vi "GMLAN InitializeConnection.vi"(0 "CAN Interface":string(combo)="CAN1", 5 "Baudrate":u32, 7 "Transmit ID":u32, 9 "Receive ID":u32, 11 "error in (no error)":errorcluster, 12 "UUDT Receive ID":u32) -> (4 "UUDT Engine":T1, 6 "ADCS Ref":T2={"Diag CAN Handle"=0, "Transport Protocol"=enum."ISO TP - Normal Mode", "Receive Address Extension"=0, "Transmit Address Extension"=0, "Receive CAN Id"=0, "Transmit CAN Id"=0, "Log Frames ?"=FALSE, "My TP Address"=0, "Other TP Address"=0, "T1"=0, "T2"=0, "T3"=0, "T4"=0, "Tx SN"=0, "Block Size"=0, "Rx SN"=0, "VW TP Initialized?"=FALSE, "Tx block no"=0, "baud rate"=0, "Interface"="", "Channel Diag CAN Handle"=0, "UDP Connection ID"=refnum, "TCP Connection ID"=refnum, "Target IP Addr"=0, "Source Address"=0, "Target Address"=0, "Send Header NACK?"=FALSE, "DLL Handle"=0, "NAD"=0, "Time Stamp read first"=0.0, "Time Stamp read last"=0.0, "Time Stamp write first"=0.0, "Time Stamp write last"=0.0, "Time Stamp write"=0.0, "Time Stamp read"=0.0, " I/O Mode"=0, "FD Baudrate"=0, "TX_DL"=8, "RX_DL"=8, "DoIP Protocol Version"=1, " Selected I/O Mode"=0, "TesterPresent Counter"=0, "TesterPresent Limit"=0, "TesterPresent Tick[ms]"=10, "TesterPresent RequireResponse?"=FALSE, "TesterPresent Stored Ref?"=FALSE, "TesterPresent Message"=[], "TesterPresent Task Handle"=0, "TesterPresent Semaphore"=refnum, "Response Plausibility Check"=1, "Default Version?"=TRUE, "Diagostic Globals"={"Timeout FC (Bs)"=250, "Timeout CF (Cr)"=250, "Timeout Diag Command"=1000, "Receive Block Size (BS)"=0, "Wait Time CF (STmin)"=5, "Max Waits (N_WFTmax)"=10, "Waits to Send (N_WAIT)"=0, "Time between Waits (TW)"=25, "Fill CAN Frames?"=TRUE, "Fill Byte"=255, "Invalid Response as Error?"=FALSE, "Max RspPending Count"=5, "VWTP Command Timeout"=50, "Transport Protocol"=enum."Diagnostics on IP", "Diag CAN Handle"=0, "DLL Handle"=0, "Timeout RspPending"=1000}, "Session-based Properties?"=FALSE} {"Diagostic Globals"."Fill Byte" format="%x"; "TesterPresent Message" format="%.0x"; "Selected I/O Mode" items=["CAN", "CAN FD", "CAN FD+BRS", "ECU Determined"]; "DoIP Protocol Version" items=["2010"=1, "2012"=2]; "RX_DL" items=["8"=8, "12"=12, "16"=16, "20"=20, "24"=24, "32"=32, "48"=48, "64"=64]; "TX_DL" items=["8"=8, "12"=12, "16"=16, "20"=20, "24"=24, "32"=32, "48"=48, "64"=64]; "I/O Mode" items=["CAN", "CAN FD", "CAN FD+BRS", "Not yet determined"]}, 15 "error out":errorcluster)   [LabVIEW 2019, in "GMLAN.lvlib"]
uses:
  GMLAN.lvlib
  <vilib>/Automotive Diagnostic Command Set/Diagnostic Transport.llb/Diag Reference.ctl
  <vilib>/Automotive Diagnostic Command Set/Diagnostic Transport.llb/Transport Protocol Selector.ctl
  <vilib>/Automotive Diagnostic Command Set/Diagnostic Transport.llb/DoIP Protocol Version.ctl
  <vilib>/Automotive Diagnostic Command Set/Diagnostic Transport.llb/Diag Globals.ctl
  _Types/UUDT Engine Refs.ctl
  _Types/UUDT Engine Connection List_Action.ctl
  <vilib>/xnet/xnet.llb/XNET Create Session (Frame Input Queued).vi
  <vilib>/addons/Automotive Diagnostic Command Set/NI_Automotive Diagnostic Command Set.lvlib
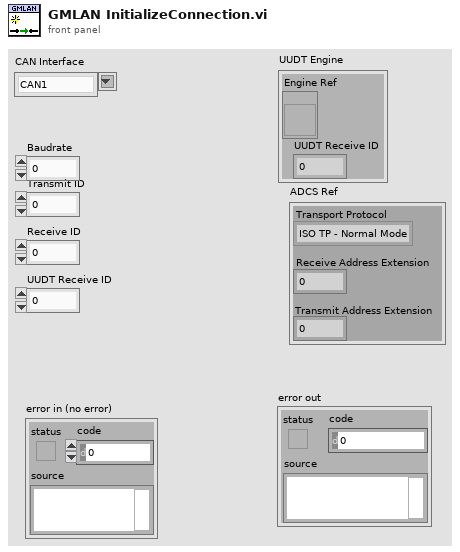
[diagram p1: front panel]
types:
  T1 = typedef "GMLAN.lvlib/UUDT Engine Refs.ctl" = cluster{"Engine Ref":refnum<vi>, "UUDT Receive ID":u32}
  T2 = typedef "NI_Automotive Diagnostic Command Set.lvlib/Diag Reference.ctl" = cluster{"Diag CAN Handle":u32, "Transport Protocol":T3, "Receive Address Extension":u8, "Transmit Address Extension":u8, "Receive CAN Id":u32, "Transmit CAN Id":u32, "Log Frames ?":bool, "My TP Address":u8, "Other TP Address":u8, "T1":u16, "T2":u16, "T3":u16, "T4":u16, "Tx SN":u8, "Block Size":u8, "Rx SN":u8, "VW TP Initialized?":bool, "Tx block no":u8, "baud rate":u64, "Interface":string, "Channel Diag CAN Handle":u32, "UDP Connection ID":refnum<k16>, "TCP Connection ID":refnum<k5>, "Target IP Addr":u32, "Source Address":u16, "Target Address":u16, "Send Header NACK?":bool, "DLL Handle":u32, "NAD":u8, "Time Stamp read first":dbl, "Time Stamp read last":dbl, "Time Stamp write first":dbl, "Time Stamp write last":dbl, "Time Stamp write":dbl, "Time Stamp read":dbl, " I/O Mode":u32, "FD Baudrate":u64, "TX_DL":u16, "RX_DL":u16, "DoIP Protocol Version":T4, " Selected I/O Mode":u32, "TesterPresent Counter":u32, "TesterPresent Limit":u32, "TesterPresent Tick[ms]":i32, "TesterPresent RequireResponse?":bool, "TesterPresent Stored Ref?":bool, "TesterPresent Message":u8[], "TesterPresent Task Handle":i32, "TesterPresent Semaphore":T5, "Response Plausibility Check":u32, "Default Version?":bool, "Diagostic Globals":T6, "Session-based Properties?":bool}
  T3 = typedef "NI_Automotive Diagnostic Command Set.lvlib/Transport Protocol Selector.ctl" = enum16{"ISO TP - Normal Mode", "ISO TP - Mixed Mode", "VW TP 2.0", "Diagnostics on IP", "ISO TP LIN"}
  T4 = typedef "NI_Automotive Diagnostic Command Set.lvlib/DoIP Protocol Version.ctl" = u8
  T5 = typedef "Semaphore RefNum" = refnum<k1>
  T6 = typedef "NI_Automotive Diagnostic Command Set.lvlib/Diag Globals.ctl" = cluster{"Timeout FC (Bs)":u32, "Timeout CF (Cr)":u32, "Timeout Diag Command":u32, "Receive Block Size (BS)":u8, "Wait Time CF (STmin)":u8, "Max Waits (N_WFTmax)":u8, "Waits to Send (N_WAIT)":i32, "Time between Waits (TW)":u32, "Fill CAN Frames?":bool, "Fill Byte":u32, "Invalid Response as Error?":bool, "Max RspPending Count":u32, "VWTP Command Timeout":u32, "Transport Protocol":T3, "Diag CAN Handle":u32, "DLL Handle":u32, "Timeout RspPending":u32}
  T7 = typedef "GMLAN.lvlib/UUDT Engine Connection List_Action.ctl" = enum8{"Initialize", "Write", "Add", "Read"}
  T8 = cluster{"Parameter Name":string, "Initial Settings":variant}
  T9 = cluster{"Frame name":string, "Identifier":u32, "Payload Length":u32, "Timing Type":u32, "Transmit Time":dbl, "Extended Identifier?":bool, "Comment":string}
  T10 = cluster{"Parameter Name":string, "Initial Settings":variant}[]
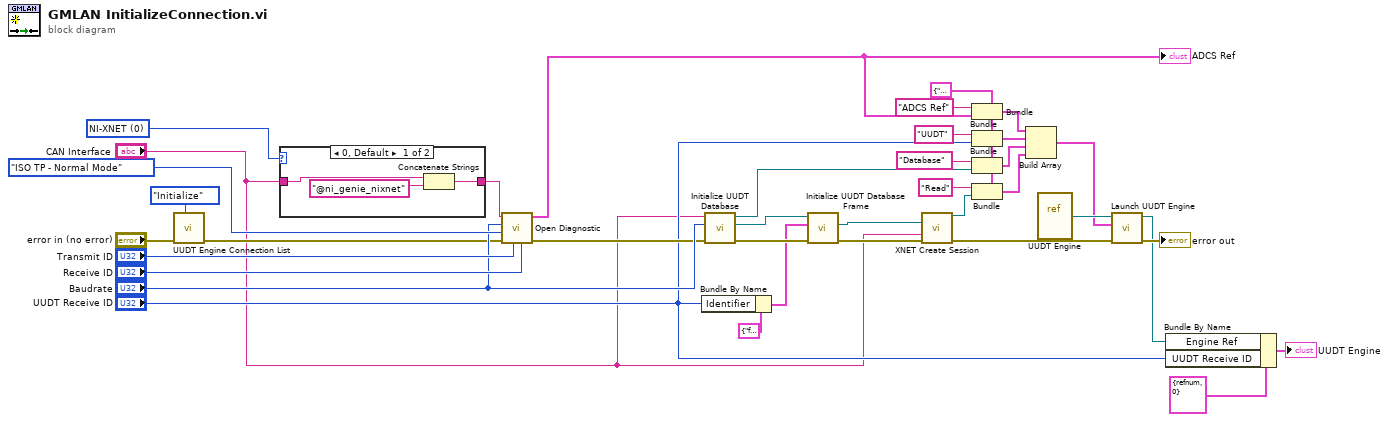
[diagram p0: block diagram]
diagram:
  w3 = u16 0 items=["NI-XNET", "NI-CAN"] ("HW select")
  w18 = T8 {"Parameter Name"="", "Initial Settings"=variant} ("Parameters")
  n1 = call "UUDT Engine Connection List.vi"("Action"=UUDT_Engine_Connection_List_Action."Initialize", "error in"="error in (no error)") -> ("error out"=w5:errorcluster)  [unwired: 8 in, 1 out]
  n2 = case shown="0, Default" w3 {
    tunnel: "CAN Interface" -> [w40 w41]
    tunnel: [w39 w41] -> w1
    frame 0, Default {
      n3 = Concatenate Strings(w40, "@ni_genie_nixnet" ("string")) -> (w39:string)
    }
    frame 1 {
    }
  }
  n4 = call <vilib>:"Open Diagnostic.vi"("Receive ID"="Receive ID", "Transmit ID"="Transmit ID", "error in (no error)"=w5, "Transport Protocol"=Transport_Protocol_Selector."ISO TP - Normal Mode", "Baud Rate"="Baudrate", "CAN Interface"=w1) -> ("error out"=w27:errorcluster, "diag ref out"=w17:T2)  [unwired: 4 out]
  "ADCS Ref" <- w17
  n5 = Bundle By Name(cluster=T9 {"Frame name"="frame1", "Identifier"=1, "Payload Length"=8, "Timing Type"=1, "Transmit Time"=0.0, "Extended Identifier?"=FALSE, "Comment"=""} ("CAN Frame"), "Identifier"="UUDT Receive ID") -> (w29:T9)
  n6 = call "Initialize UUDT Database.vi"("error in (no error)"=w27, "Baud Rate"="Baudrate", "Addon Name"="CAN Interface") -> ("error out"=w34:errorcluster, "Cluster"=w33:refnum<k21>, "XNET Database"=w19:refnum<k21>)  [unwired: 6 in]
  n7 = call "Initialize UUDT Database Frame.vi"("error in"=w34, "CAN Frame"=w29, "cluster in"=w33) -> ("error out"=w31:errorcluster, "frame out"=w32:refnum<k21>)  [unwired: 6 in, 1 out]
  n8 = call-poly <vilib>:"XNET Create Session.vi"("frame"=w32, "interface"="CAN Interface", "error in (no error)"=w31) -> ("session out"=w21:refnum<k21>, "error out"=w26:errorcluster)  [unwired: 11 out]
  n9 = Bundle(cluster=w18, "Parameter Name"="ADCS Ref", "Initial Settings"=w17) -> (w15:T8)
  n10 = Bundle(cluster=w18, "Parameter Name"="UUDT", "Initial Settings"="UUDT Receive ID") -> (w14:T8)
  n11 = Bundle(cluster=w18, "Parameter Name"="Database", "Initial Settings"=w19) -> (w13:T8)
  n12 = Bundle(cluster=w18, "Parameter Name"="Read", "Initial Settings"=w21) -> (w12:T8)
  n13 = Build Array(w15, w14, w13, w12) -> (w11:T10)
  n14 = vi-ref "UUDT Engine.vi"() -> (w24:refnum<vi>)
  n15 = call "Launch UUDT Engine.vi"("error in (no error)"=w26, "Initial Parameters"=w11, "VI Ref In"=w24) -> ("error out"=→"error out":errorcluster, "VI Ref Out"=w10:refnum<vi>)  [unwired: 7 in]
  n16 = Bundle By Name(cluster=T1 {"Engine Ref"=refnum, "UUDT Receive ID"=0} ("UUDT Engine"), "Engine Ref"=w10, "UUDT Receive ID"="UUDT Receive ID") -> (→"UUDT Engine":T1)
